vi "scale.vi"(0 "reference":refnum<class "Graphics.lvclass">, 1 "scaleX":dbl=1.0 format="%.2f", 2 "scaleY":dbl=1.0 format="%.2f", 5 "error in (no error)":errorcluster) -> (14 "reference out":refnum<class "Graphics.lvclass">, 19 "error out":errorcluster)   [LabVIEW 2012, in "Graphics.lvclass"]
doc: "Scale (x,y)\n1 is default\nMust be bigger than 0"
uses:
  <resource>/Framework/Providers/Open_GDS/UML/Graphics_class/Graphics.lvclass
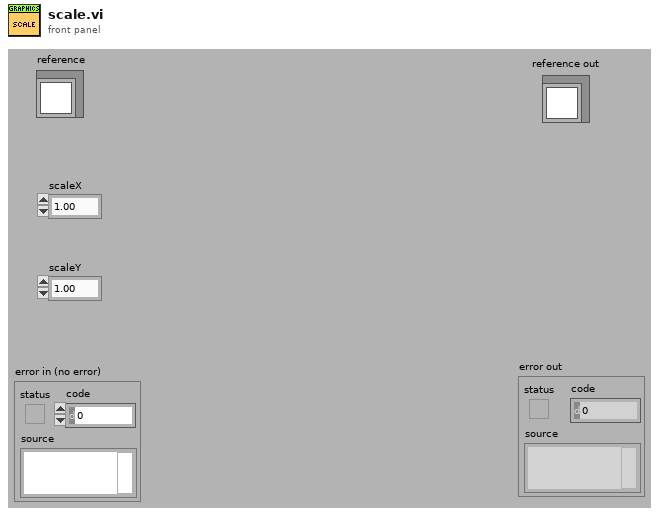
[diagram p1: front panel]
types:
  T1 = typedef "Graphics.lvclass/ObjectAttributes.ctl" = cluster{"drawColor":u32, "backgroundColor":u32, "font":T2, "fontType":T3, "picture":picture, "stroke":T4, "scaleX":dbl, "scaleY":dbl, "screenRef":refnum<vi>, "offsetX":dbl, "offsetY":dbl}
  T2 = typedef "Graphics.lvclass/FontType.ctl" = cluster{"Font Name:":string, "Size":i16, "Strikeout?":bool, "Italic?":bool, "Underline?":bool, "Outline?":bool, "Shadow?":bool, "Bold?":bool}
  T3 = typedef "Graphics.lvclass/LvFontType.ctl" = enum16{"User-specified Font", "Application Font", "System Font", "Dialog Font"}
  T4 = typedef "Graphics.lvclass/StrokeType.ctl" = enum16{"USE_DEFAULT", "SOLID", "DOTTED"}
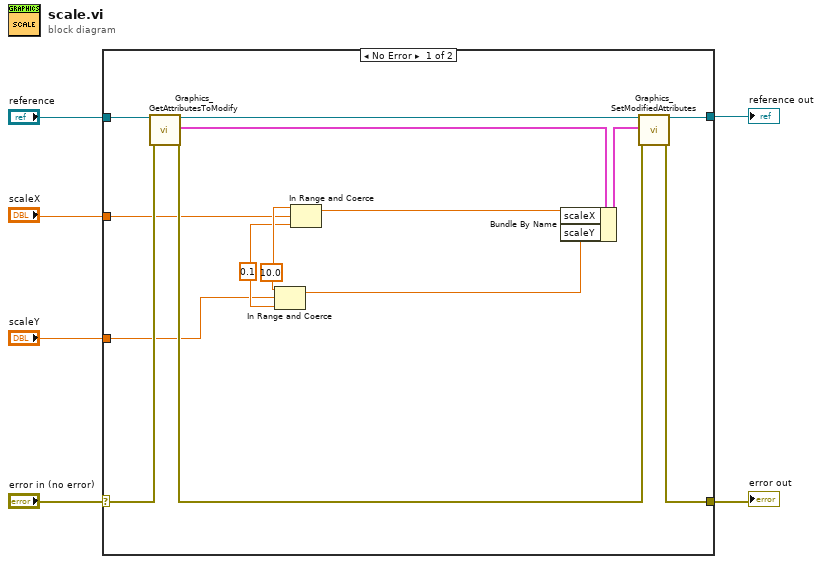
[diagram p0: block diagram]
diagram:
  n1 = case shown="No Error" "error in (no error)" {
    selector: "error in (no error)" -> [w20 w21]
    tunnel: "reference" -> [w19 w22]
    tunnel: [w14 w21] -> w4
    tunnel: [w13 w22] -> w3
    tunnel: "scaleX" -> [w10 _]
    tunnel: "scaleY" -> [w9 _]
    frame No Error {
      w12 = 10.0 ("upper limit")
      w11 = 0.1 ("lower limit")
      n2 = call <resource>:"Graphics_GetAttributesToModify.vi"("reference in"=w19, "error in (no error)"=w20) -> ("reference out"=w17:refnum<class "Graphics.lvclass">, "Attributes"=w16:T1, "error out"=w18:errorcluster)  [unwired: 1 in, 14 out]
      n3 = In Range and Coerce(upper limit=w12, x=w9, lower limit=w11) -> (coerced(x)=w8:dbl)  [unwired: 1 out]
      n4 = In Range and Coerce(upper limit=w12, x=w10, lower limit=w11) -> (coerced(x)=w7:dbl)  [unwired: 1 out]
      n5 = Bundle By Name(cluster=w16, "scaleX"=w7, "scaleY"=w8) -> (w15:T1)
      n6 = call <resource>:"Graphics_SetModifiedAttributes.vi"("reference in"=w17, "Attributes"=w15, "error in (no error)"=w18) -> ("reference out"=w13:refnum<class "Graphics.lvclass">, "error out"=w14:errorcluster)  [unwired: 3 in, 12 out]
    }
    frame Error {
    }
  }
  "reference out" <- w3
  "error out" <- w4
